vi "Run.vi"(8 "error in":errorcluster, 9 "Actor-Event-Registrations":T2, 10 "Actor-Events":T1, 11 "Actor in":refnum<class "Copy of Actor.lvclass">) -> (0 "error out":errorcluster, 3 "Actor out":refnum<class "Copy of Actor.lvclass">)   [LabVIEW 2018, in "Copy of Actor.lvclass"]
uses:
  Copy of Actor.lvclass
  Event-Registrations.ctl
  Stop.ctl
  Event-References.ctl
  Launched.ctl
  Some Request.ctl
  Some Response.ctl
  Initialize Event References.vi
  Initialize Event Registrations.vi
types:
  T1 = typedef "Copy of Actor.lvclass/Event-References.ctl" = cluster{"Stop":refnum<user-event>, "Launched":refnum<user-event>, "Some Request":refnum<user-event>}
  T2 = typedef "Copy of Actor.lvclass/Event-Registrations.ctl" = cluster{"Stop":refnum<event-registration>}
  T3 = typedef "Copy of Actor.lvclass/Launched.ctl" = cluster{"Launched State":refnum<class "Copy of Actor.lvclass">}
  T4 = typedef "Copy of Actor.lvclass/Stop.ctl" = enum16{"Normal", "Emergency"}
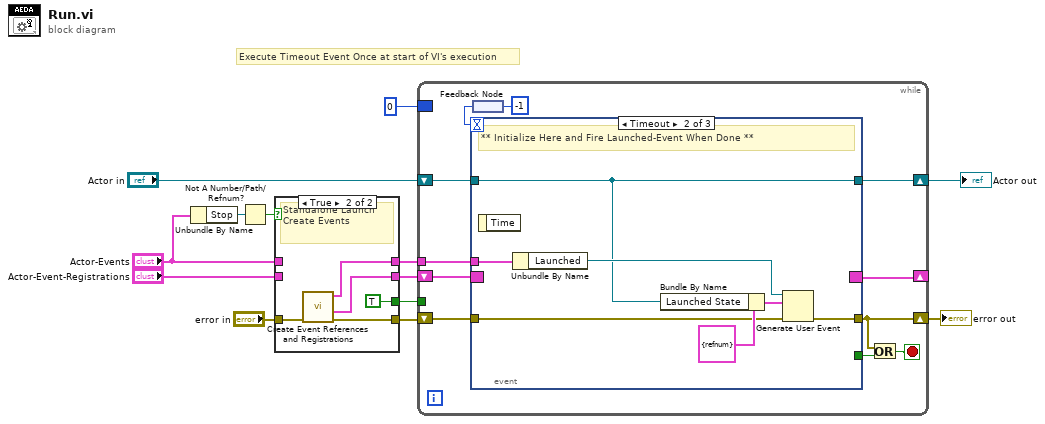
[diagram p0: block diagram]
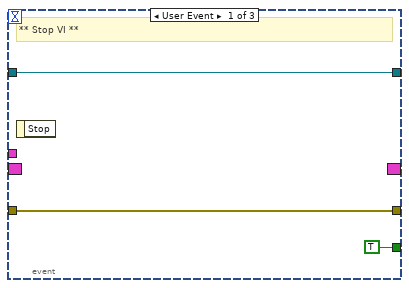
[diagram p2: hidden frame]
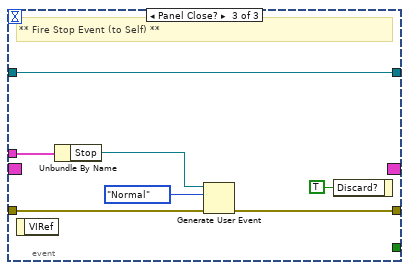
[diagram p3: hidden frame]
diagram:
  # "Execute Timeout Event Once at start of VI's execution"
  n1 = Unbundle By Name("Actor-Events") -> ("Stop"=w5:refnum<user-event>)
  n2 = Not A Number/Path/Refnum?(number/path/refnum=w5) -> (NaN/Path/Refnum?=w4:bool)
  n3 = case shown="True" w4 {
    tunnel: "Actor-Events" -> [w16 _]
    tunnel: "Actor-Event-Registrations" -> [w15 _]
    tunnel: "error in" -> [w14 w21]
    tunnel: [w14 w20] -> w7
    tunnel: [w15 w18] -> w3
    tunnel: [w16 w19] -> w2
    tunnel: [_ TRUE] -> w1
    frame False {
      # "External Launch\nEvents Already Exist"
    }
    frame True {
      # "Standalone Launch\nCreate Events"
      n4 = call "Create Event References and Registrations.vi"("error in (no error)"=w21) -> ("error out"=w20:errorcluster, "Event-Registrations"=w18:T2, "Event-References"=w19:T1)  [unwired: 8 in]
    }
  }
  n5 = while {
    shift-right: [w29] -> w11
    shift-left: "Actor in" -> [w32]
    shift-right: [w28] -> w10
    shift-left: w7 -> [w31]
    shift-right: [w30] -> _
    shift-left: w3 -> [w22]
    border: 0 -> [_]
    tunnel: w2 -> [w23]
    tunnel: w1 -> [_]
    stop <- w26 stop-if-true
    n6 = feedback #1() -> (w24:i32)
    n7 = event shown="[1] Timeout" {
      selector: w22 -> [_ _ _]
      dyn-events: [_ _ _] -> w30
      timeout: w24 -> [_ _ _]
      tunnel: w32 -> [w35 w36 w48]
      tunnel: w31 -> [w34 w40 w47]
      tunnel: [w35 w36 w48] -> w29
      tunnel: [w34 w39 w46] -> w28
      tunnel: [TRUE _ _] -> w27
      tunnel: w23 -> [_ w38 w44]
      event User Event {
        # "** Stop VI **"
        n8 = event-data() -> ()  [unwired: 1 in, 1 out]
      }
      event Timeout {
        # "** Initialize Here and Fire Launched-Event When Done **"
        n9 = event-data() -> ()  [unwired: 1 in, 1 out]
        n10 = Unbundle By Name(w38) -> ("Launched"=w37:refnum<user-event>)
        n11 = Bundle By Name(cluster=T3 {"Launched State"=refnum} ("event data"), "Launched State"=w36) -> (w41:T3)
        n12 = Generate User Event(user event=w37, event data cluster=w41, error in=w40) -> (error out=w39:errorcluster)  [unwired: 1 in, 1 out]
      }
      event Panel Close? {
        # "** Fire Stop Event (to Self) **"
        n13 = event-data() -> ()  [unwired: 1 in, 1 out]
        n14 = Unbundle By Name(w44) -> ("Stop"=w43:refnum<user-event>)
        n15 = Generate User Event(user event=w43, event data cluster=Stop."Normal" ("event data"), error in=w47) -> (error out=w46:errorcluster)  [unwired: 1 in, 1 out]
        n16 = event-data("Discard?"=TRUE) -> ()  [unwired: 1 in, 1 out]
      }
    }
    n17 = feedback-in #1(-1) -> ()
    n18 = Or(x=w28, y=w27) -> (x .or. y?=w26:bool)
  }
  "error out" <- w10
  "Actor out" <- w11
